vi "H5Pcreate.vi"(6 "error in (no error)":errorcluster, 9 "Property List Class":T1=enum."H5P_FILE_CREATE") -> (0 "error out":errorcluster, 3 "HDF5 Property List Ref":T2)   [LabVIEW 2017]
doc: "Creates a new property list as an instance of a property list class."
uses:
  <vilib>/UPVI/lvhdf5/library.llb/HDF5 Ref.ctl
  <vilib>/UPVI/lvhdf5/property.llb/LVH5PClassId.ctl
  <vilib>/UPVI/lvhdf5/hdf5.dll
panel:
  # "LVHDF5 Toolkit\nCopyright (c) 2005-2013 by Jason D. Sommerville\nCopyright (c) 2014 by UPVI, LLC.\n\nThis use and distribution of this file is governed by the terms found in \nLICENSE.txt distributed with this toolkit and installed at\n <user.lib>\\_lvhdf5\\LICENSE.txt"
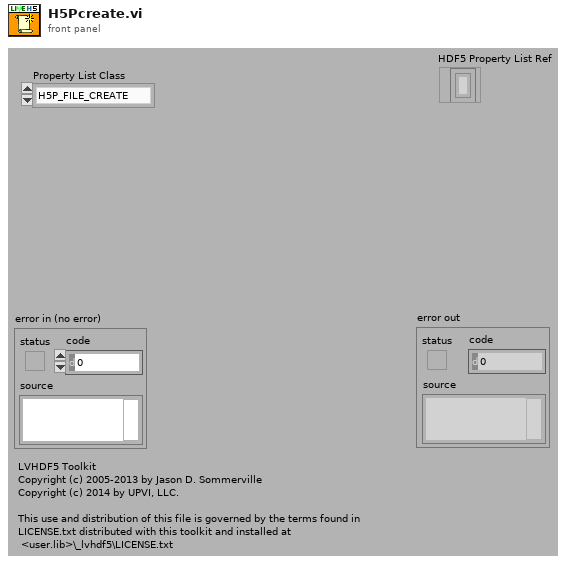
[diagram p1: front panel]
types:
  T1 = typedef "LVH5PClassId.ctl" = enum32{"H5P_ROOT", "H5P_OBJECT_CREATE", "H5P_FILE_CREATE", "H5P_FILE_ACCESS", "H5P_DATASET_CREATE", "H5P_DATASET_ACCESS", "H5P_DATASET_XFER", "H5P_FILE_MOUNT", "H5P_GROUP_CREATE", "H5P_GROUP_ACCESS", "H5P_DATATYPE_CREATE", "H5P_DATATYPE_ACCESS", "H5P_STRING_CREATE", "H5P_ATTRIBUTE_CREATE", "H5P_OBJECT_COPY", "H5P_LINK_CREATE", "H5P_LINK_ACCESS"}
  T2 = typedef "HDF5 Ref.ctl" = refnum<k1>
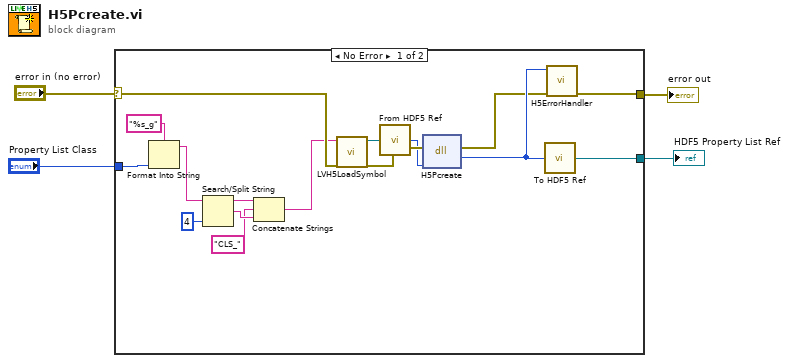
[diagram p0: block diagram]
diagram:
  n1 = case shown="No Error" "error in (no error)" {
    selector: "error in (no error)" -> [w15 w21]
    tunnel: [w20 w21] -> w3
    tunnel: "Property List Class" -> [w16 _]
    tunnel: [w18 _] -> w1
    frame No Error {
      n2 = Format Into String(format string="%s_g", w16) -> (resulting string=w10:string)  [unwired: 2 in, 1 out]
      n3 = Search/Split String(string=w10, offset (0)=4) -> (substring before match=w8:string, match + rest of string=w7:string)  [unwired: 1 in, 1 out]
      n4 = Concatenate Strings(w8, "CLS_" ("string"), w7) -> (w5:string)
      n5 = call <vilib>:"LVH5LoadSymbol.vi"("error in (no error)"=w15, "Symbol"=w5) -> ("error out"=w14:errorcluster, "Refnum out"=w12:T2)  [unwired: 8 in]
      n6 = call <vilib>:"From HDF5 Ref.vi"("HDF5 Ref"=w12) -> ("I32"=w11:i32)
      n7 = dll-call lib="C:/Program Files/National Instruments/LabVIEW 2017/vi.lib/UPVI/lvhdf5/hdf5.dll" fn="H5Pcreate"(error in=w14, "cls_id"=w11) -> (error out=w13:errorcluster, w19:i32)  [unwired: 3 in, 1 out]
      n8 = call <vilib>:"To HDF5 Ref.vi"("I32"=w19) -> ("HDF5 Ref"=w18:T2)
      n9 = call <vilib>:"H5ErrorHandler.vi"("error in (no error)"=w13, "herr_t"=w19) -> ("error out"=w20:errorcluster)  [unwired: 3 in, 4 out]
    }
    frame Error {
    }
  }
  "error out" <- w3
  "HDF5 Property List Ref" <- w1
